vi "Process.vi"(8 "error in":errorcluster, 11 "Example Instrument":refnum<class "Example Instrument.lvclass">) -> (0 "error out":errorcluster, 3 "Example Instrument out":refnum<class "Example Instrument.lvclass">)   [LabVIEW 2016, in "Example Instrument.lvclass"]
doc: "---------------------------------------------------------------\nJKI State Machine Objects™\nhttp://jki.net/state-machine-objects/\nCopyright (C) 2005-2015, JKI <info@jki.net>\nALL RIGHTS RESERVED"
uses:
  Example Instrument.lvclass
  C:/Program Files (x86)/National Instruments/LabVIEW 2016/vi.lib/JKI/JKI SMO/SMO/SMO.lvclass
  <vilib>/JKI/JKI SMO/SMO/Typedefs/Parent Call--Enum.ctl
  Typedefs/PrivateEvents--Example Instrument.setMagnet.ctl
  RemoteControl/RemoteControl.lvclass
  Instrument/Instrument.lvclass
  <vilib>/JKI/JKI SMO/SMO/SMO.lvclass
panel:
  # "Example INSTRUMENT"
  # "For instructions on how to use the JKI State Machine Objects, examples and video tutorials, visit:\nhttp://jki.net/state-machine-objects/\n\nJKI State Machine Objects™\nhttp://jki.net/state-machine-objects/\nCopyright (C) 2005-2015, JKI <info@jki.net>\nALL RIGHTS RESERVED"
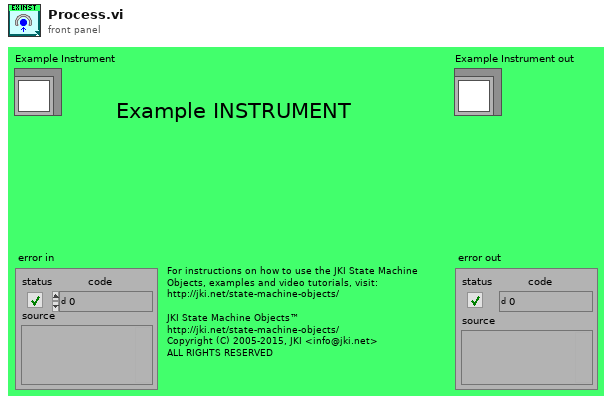
[diagram p1: front panel]
types:
  T1 = typedef "SMO.lvclass/Parent Call--Enum.ctl" = enum16{"Allows parent to run", "Does not request parent to run"}
  T2 = enum32{"invalid app kind", "Development System", "Run Time System", "Student Edition", "Embedded LabVIEW", "Evaluation", "Custom"}
  T3 = enum32{"Invalid", "Standard", "Closed", "Hidden", "Minimized", "Maximized"}
  T4 = enum32{"Bad", "Idle", "Run top level", "Running"}
  T5 = typedef "Example Instrument.lvclass/PrivateEvents--Example Instrument.setMagnet.ctl" = cluster{"setMagnet":dbl, "notifier":refnum<notifier>}
  T6 = cluster{"Core":cluster{"Current VI Reference":refnum<vi>, "Close Panel on Exit?":bool, "error":errorcluster}, "Self Reference":refnum<class "Example Instrument.lvclass">, "setMagnet":T5, "RemoteControl.lvclass":refnum<class "RemoteControl.lvclass">}
  T7 = cluster{"Current VI Reference":refnum<vi>, "Close Panel on Exit?":bool, "error":errorcluster}
  T8 = typedef "SMO.lvclass/Protected Events.ctl" = cluster{"StopProcesses":refnum<user-event>, "AbortProcesses":refnum<user-event>, "Config Changed":refnum<user-event>, "Dependency":refnum<user-event>}
  T9 = typedef "Example Instrument.lvclass/PrivateEvents--Cluster.ctl" = cluster{"setMagnet":refnum<user-event>}
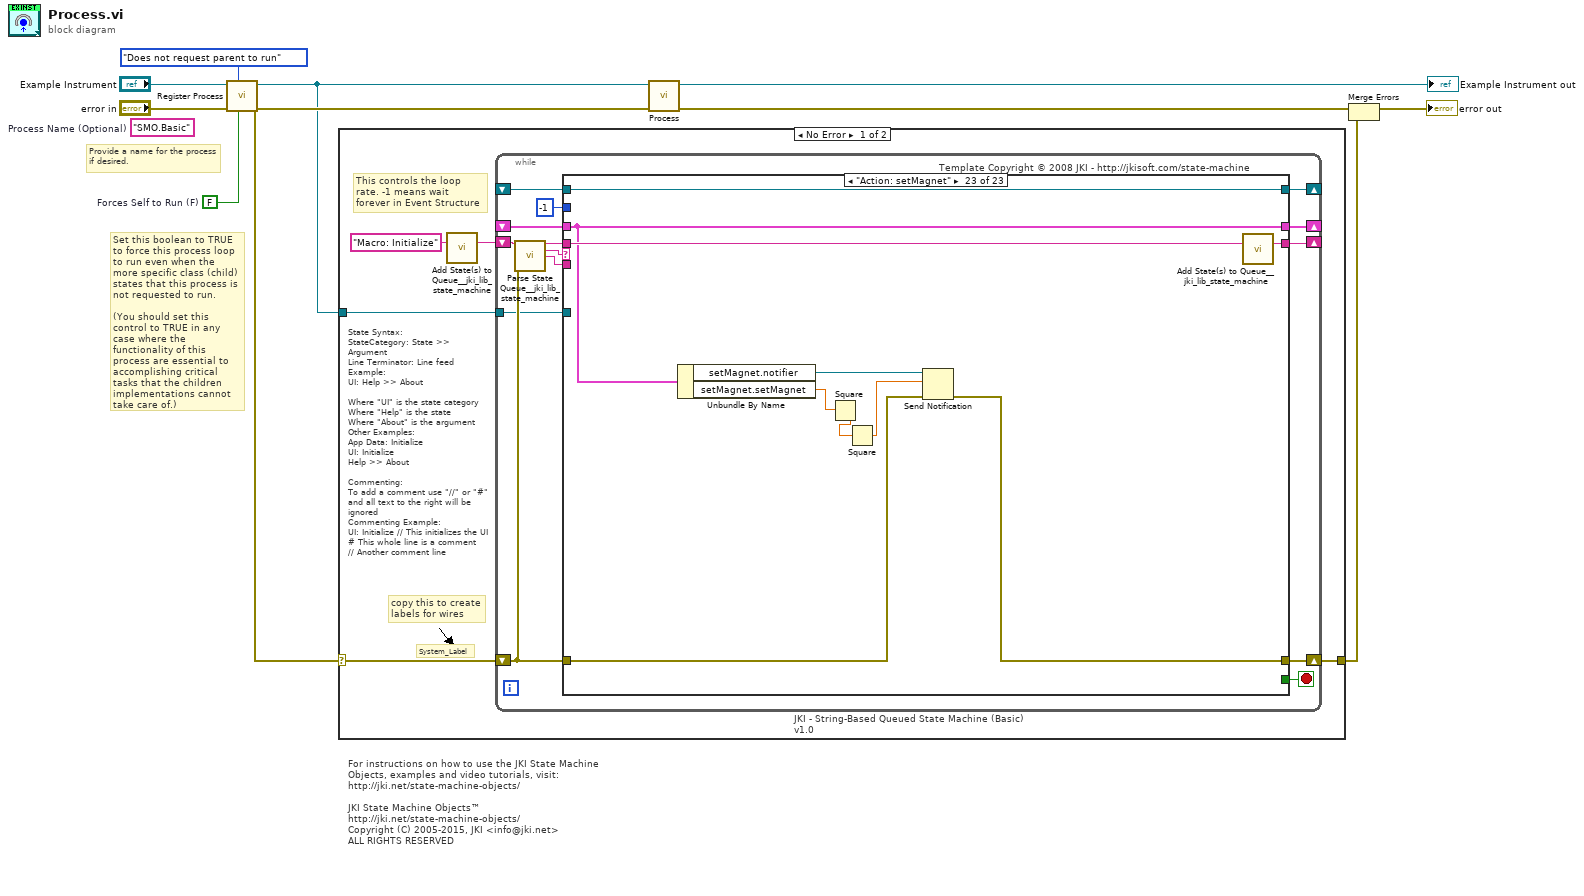
[diagram p0: block diagram]
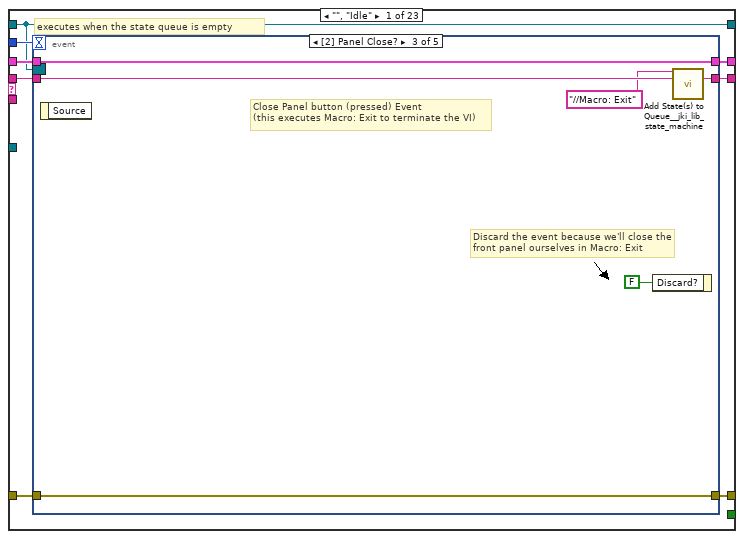
[diagram p2: hidden frame]
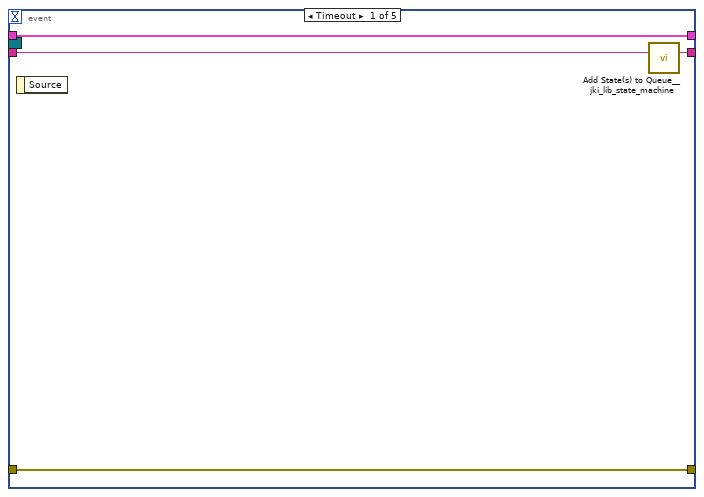
[diagram p3: hidden frame]
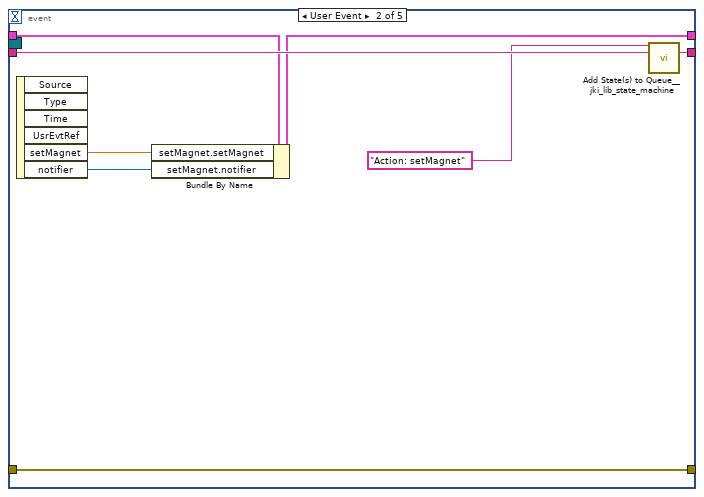
[diagram p4: hidden frame]
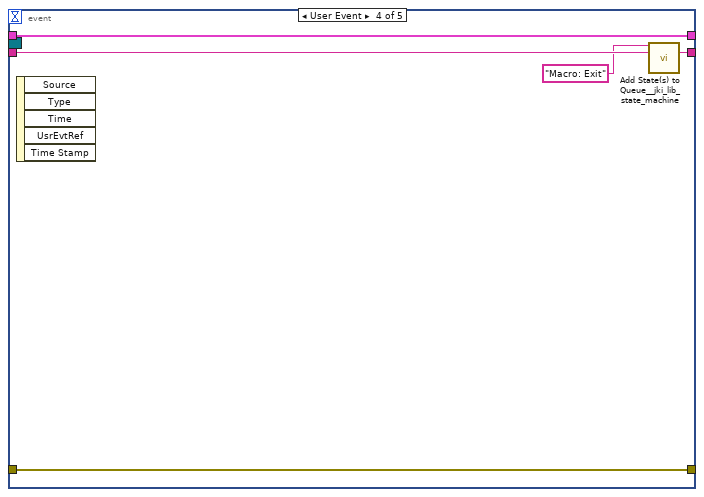
[diagram p5: hidden frame]
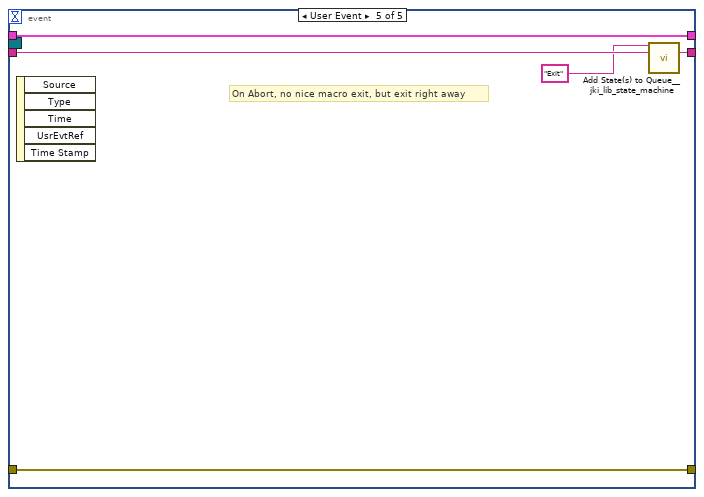
[diagram p6: hidden frame]
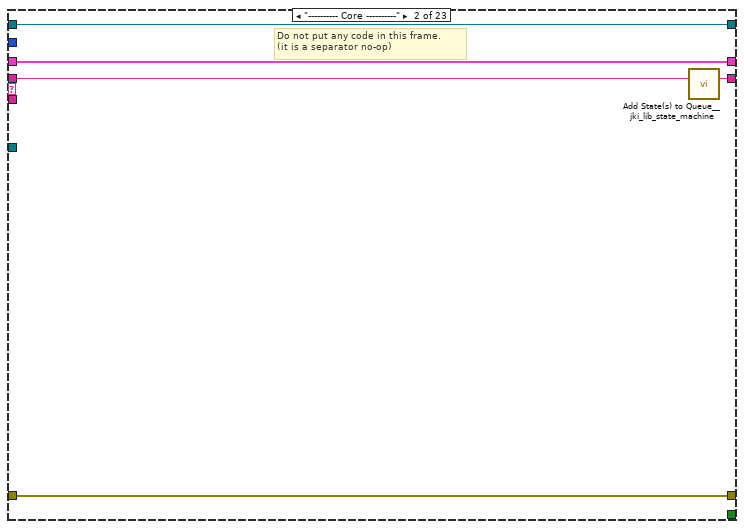
[diagram p7: hidden frame]
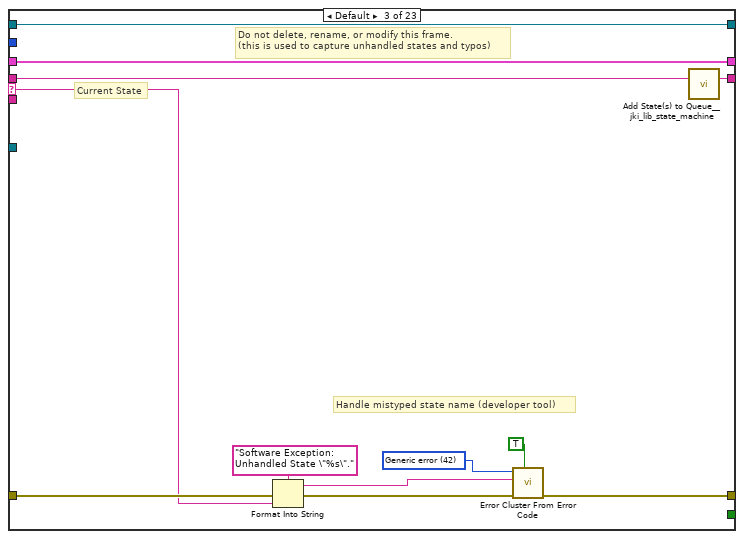
[diagram p8: hidden frame]
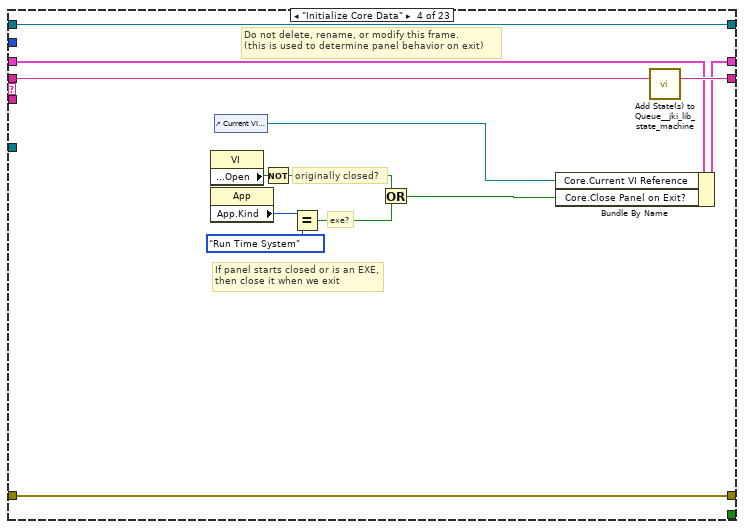
[diagram p9: hidden frame]
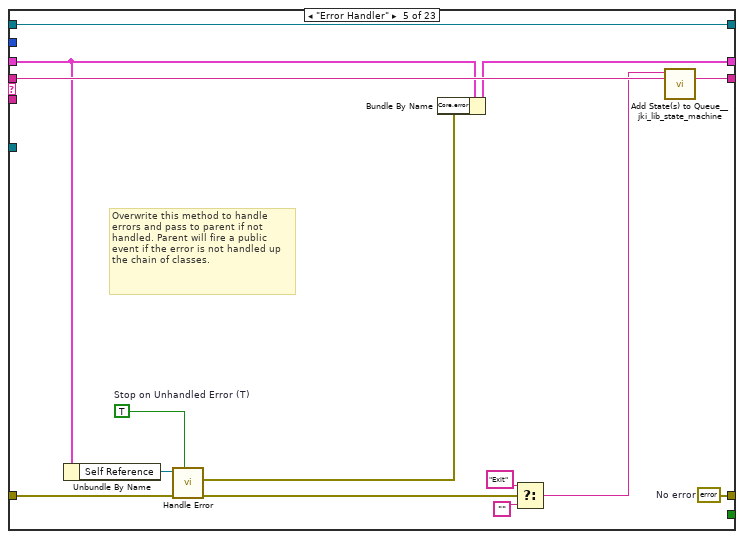
[diagram p10: hidden frame]
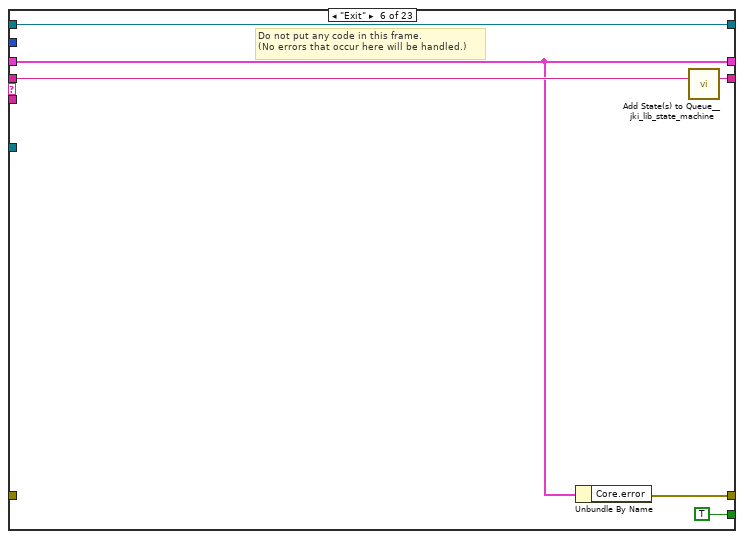
[diagram p11: hidden frame]
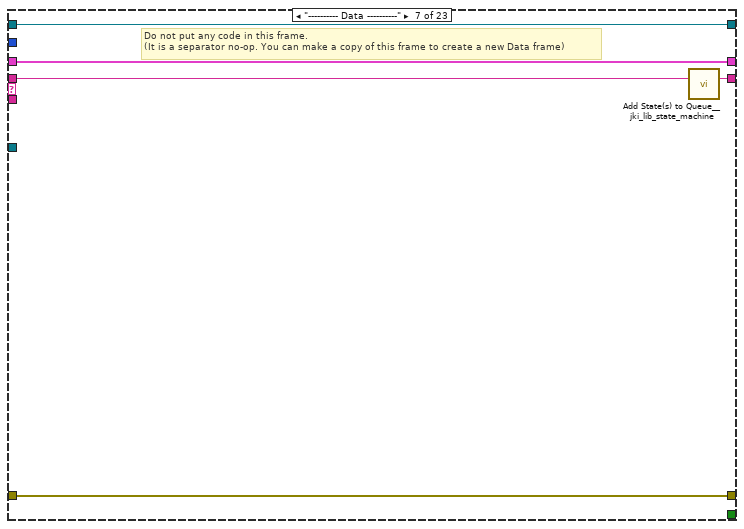
[diagram p12: hidden frame]
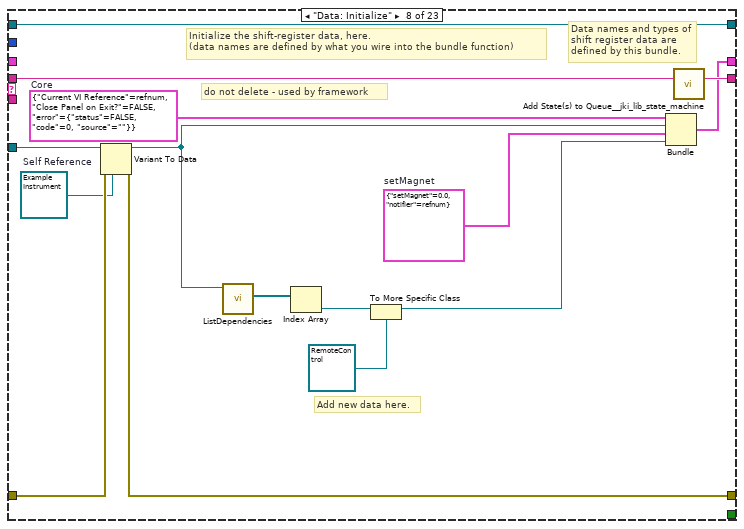
[diagram p13: hidden frame]
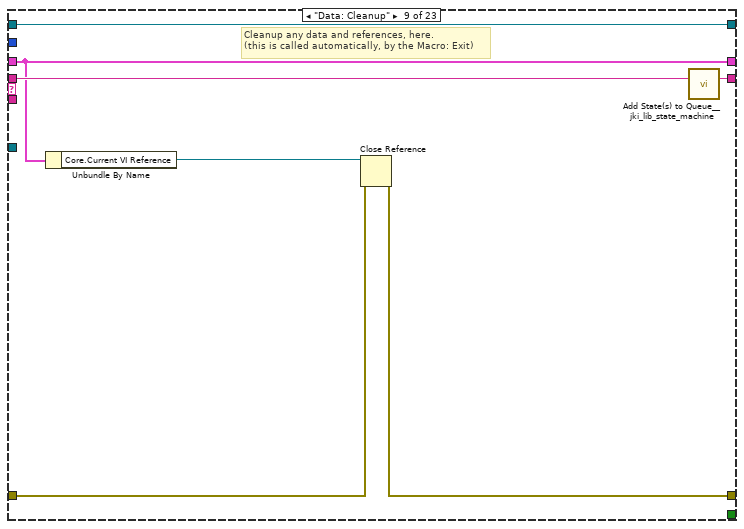
[diagram p14: hidden frame]
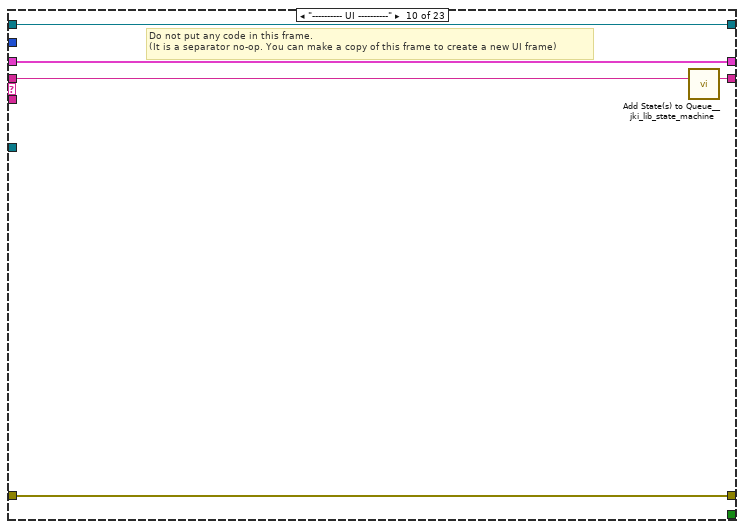
[diagram p15: hidden frame]
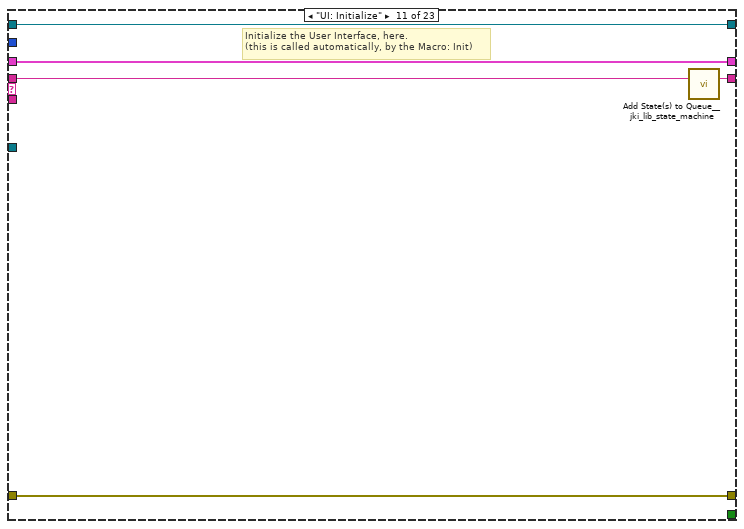
[diagram p16: hidden frame]
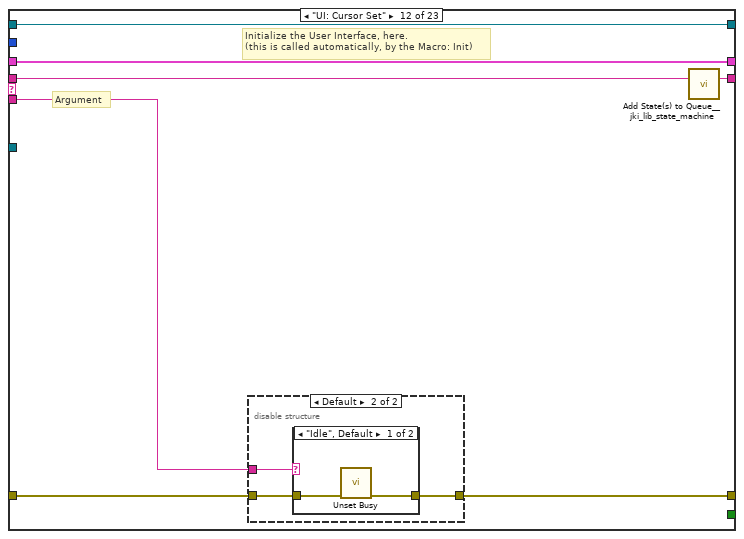
[diagram p17: hidden frame]
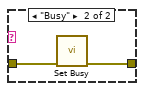
[diagram p19: hidden frame]
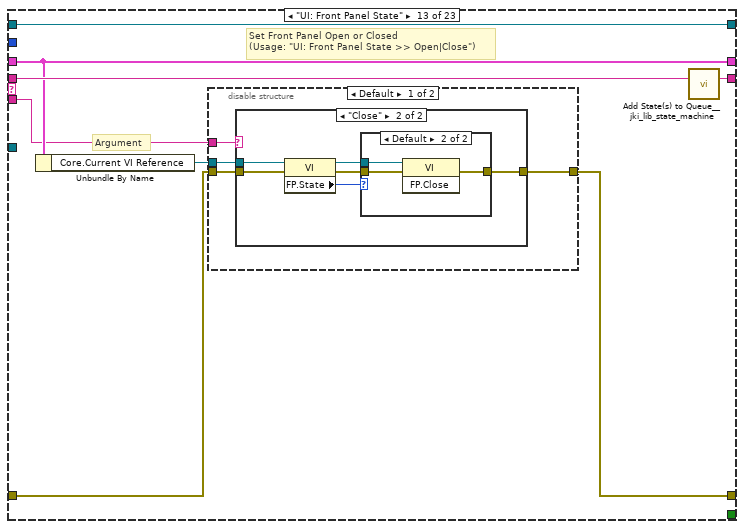
[diagram p20: hidden frame]
diagram:
  w1 = FALSE  # Forces Self to Run (F)
  (unwired) "SMO.Basic"  # Process Name (Optional)
  # "Provide a name for the process\nif desired."
  # "Set this boolean to TRUE to force this process loop to run even when the more specific class (child) states that this process is not requested to run.\n\n(You should set this control to TRUE in any case where the functionality of this process are essential to accomplishing critical tasks that the children implementations cannot take care of.)"
  # "For instructions on how to use the JKI State Machine Objects, examples and video tutorials, visit:\nhttp://jki.net/state-machine-objects/\n\nJKI State Machine Objects™\nhttp://jki.net/state-machine-objects/\nCopyright (C) 2005-2015, JKI <info@jki.net>\nALL RIGHTS RESERVED"
  n1 = call <vilib>:"Register Process.vi"("Forces Self to Run (F)"=w1, "Parent Call"=Parent_Call--Enum."Does not request parent to run", "error in (no error)"="error in", "SMO"="Example Instrument") -> ("error out"=w7:errorcluster, "SMO out"=w6:refnum<class "Example Instrument.lvclass">)  [unwired: 6 in]
  n2 = case shown="No Error" w7 {
    selector: w7 -> [w12 w289]
    tunnel: w6 -> [w13 _]
    tunnel: [w11 w289] -> w3
    frame No Error {
      # "State Syntax:\nStateCategory: State >> Argument\nLine Terminator: Line feed\nExample:\nUI: Help >> About\n\nWhere \"UI\" is the state category\nWhere \"Help\" is the state\nWhere \"About\" is the argument\nOther Examples:\nApp Data: Initialize\nUI: Initialize\nHelp >> About\n\nCommenting:\nTo add a comment use \"//\" or \"#\" and all text to the right will be ignored\nCommenting Example:\nUI: Initialize // This initializes the UI\n# This whole line is a comment\n// Another comment line"
      # "copy this to create labels for wires"
      # "This controls the loop rate. -1 means wait forever in Event Structure"
      # "System_Label"
      n3 = call <vilib>:"Add State(s) to Queue__jki_lib_state_machine.vi"("State(s) in (\"\")"="Macro: Initialize") -> ("States Out"=w15:string)  [unwired: 14 in]
      n4 = while "JKI - String-Based Queued State Machine (Basic) v1.0" {
        shift-right: [w22] -> _
        shift-left: _ -> [w21]
        shift-right: [w25] -> w11
        shift-left: w12 -> [w19]
        shift-right: [w24] -> _
        shift-left: w15 -> [w26]
        tunnel: w13 -> [w18]
        shift-right: [w17] -> _
        shift-left: _ -> [w16]
        stop <- w23 stop-if-true
        # "Template Copyright © 2008 JKI - http://jkisoft.com/state-machine"
        n5 = call <vilib>:"Parse State Queue__jki_lib_state_machine.vi"("State Queue"=w26, "Error In (no error)"=w19) -> ("Remaining States"=w28:string, "Current State"=w29:string, "Arguments"=w27:string)  [unwired: 11 in]
        n6 = case shown="\"Action: setMagnet\"" w29 {
          selector: w29 -> [_ _ w72 _ _ _ _ _ _ _ _ _ _ _ _ _ _ _ _ _ _ _ _]
          tunnel: w28 -> [w37 w70 w76 w95 w109 w115 w120 w135 w142 w147 w152 w159 w175 w207 w221 w235 w240 w251 w256 w267 w273 w278 w288]
          tunnel: w27 -> [_ _ _ _ _ _ _ _ _ _ _ w153 w169 _ _ _ _ _ _ _ _ _ _]
          tunnel: w21 -> [w35 w67 w74 w86 w103 w111 w117 _ w137 w144 w150 w157 w171 w204 w217 w226 w237 w248 w253 w257 w271 w276 w285]
          tunnel: [w34 w68 w78 w92 w104 w110 w118 w131 w138 w145 w149 w154 w172 w205 w219 w233 w238 w242 w254 w262 w269 w274 w282] -> w25
          tunnel: w19 -> [w33 w68 w77 w92 w105 _ w118 w132 w139 w145 w149 w155 w173 w205 w219 w233 w238 w243 w254 w263 w269 w274 w283]
          tunnel: [w36 w69 w75 w94 w108 w114 w119 w134 w141 w146 w151 w158 w174 w206 w220 w234 w239 w250 w255 w266 w272 w277 w287] -> w24
          tunnel: [_ _ _ _ _ TRUE _ _ _ _ _ _ _ _ _ _ _ _ _ _ _ _ _] -> w23
          tunnel: [w32 w67 w74 w93 w102 w111 w117 w133 w137 w144 w150 w157 w171 w204 w217 w226 w237 w248 w253 w257 w271 w276 w285] -> w22
          tunnel: -1 ("Timeout") -> [w31 _ _ _ _ _ _ _ _ _ _ _ _ _ _ _ _ _ _ _ _ _ _]
          tunnel: w18 -> [_ _ _ _ _ _ _ w129 _ _ _ _ _ _ _ _ _ _ _ _ _ _ _]
          tunnel: [w30 w66 w71 w83 w107 w112 w116 w128 w136 w143 w148 w156 w168 w203 w218 w227 w236 w249 w252 w265 w270 w275 w286] -> w17
          tunnel: w16 -> [w30 w66 w71 w83 w107 w112 w116 w128 w136 w143 w148 w156 w168 w203 w218 w227 w236 w249 w252 _ w270 w275 w286]
          frame "", "Idle" {
            # "executes when the state queue is empty"
            n7 = event shown="[2] Panel Close?" {
              selector: w30 -> [_ _ _ _ _]
              dyn-events: _ -> [_ _ _ _ _]
              timeout: w31 -> [_ _ _ _ _]
              tunnel: w37 -> [w41 w49 w55 w60 w65]
              tunnel: [w40 w48 w54 w59 w64] -> w36
              tunnel: w35 -> [w38 w43 w52 w57 w62]
              tunnel: [w39 w47 w53 w58 w63] -> w34
              tunnel: w33 -> [w39 w47 w53 w58 w63]
              tunnel: [w38 w42 w52 w57 w62] -> w32
              event Timeout {
                n8 = event-data() -> ()  [unwired: 1 in, 1 out]
                n9 = call <vilib>:"Add State(s) to Queue__jki_lib_state_machine.vi"("State(s) in (\"\")"=w41) -> ("States Out"=w40:string)  [unwired: 14 in]
              }
              event User Event {
                n10 = event-data() -> ("setMagnet"=w45:dbl, "notifier"=w44:refnum<notifier>)  [unwired: 1 in, 4 out]
                n11 = Bundle By Name(cluster=w43, "setMagnet.setMagnet"=w45, "setMagnet.notifier"=w44) -> (w42:T6)
                n12 = call <vilib>:"Add State(s) to Queue__jki_lib_state_machine.vi"("State(s) in Front (\"\")"="Action: setMagnet" ("State(s) in Front (\"\")"), "State(s) in (\"\")"=w49) -> ("States Out"=w48:string)  [unwired: 13 in]
              }
              event Panel Close? {
                # "Discard the event because we'll close the front panel ourselves in Macro: Exit"
                # "Close Panel button (pressed) Event\n(this executes Macro: Exit to terminate the VI)"
                n13 = event-data() -> ()  [unwired: 1 in, 1 out]
                n14 = event-data("Discard?"=FALSE) -> ()  [unwired: 1 in, 1 out]
                n15 = call <vilib>:"Add State(s) to Queue__jki_lib_state_machine.vi"("State(s) in Front (\"\")"="//Macro: Exit", "State(s) in (\"\")"=w55) -> ("States Out"=w54:string)  [unwired: 13 in]
              }
              event User Event {
                n16 = event-data() -> ()  [unwired: 1 in, 5 out]
                n17 = call <vilib>:"Add State(s) to Queue__jki_lib_state_machine.vi"("State(s) in Front (\"\")"="Macro: Exit", "State(s) in (\"\")"=w60) -> ("States Out"=w59:string)  [unwired: 13 in]
              }
              event User Event {
                # "On Abort, no nice macro exit, but exit right away"
                n18 = event-data() -> ()  [unwired: 1 in, 5 out]
                n19 = call <vilib>:"Add State(s) to Queue__jki_lib_state_machine.vi"("State(s) in Front (\"\")"="Exit", "State(s) in (\"\")"=w65) -> ("States Out"=w64:string)  [unwired: 13 in]
              }
            }
          }
          frame "---------- Core ----------" {
            # "Do not put any code in this frame.\n(it is a separator no-op)"
            n20 = call <vilib>:"Add State(s) to Queue__jki_lib_state_machine.vi"("State(s) in (\"\")"=w70) -> ("States Out"=w69:string)  [unwired: 14 in]
          }
          frame Default {
            w81 = 42 items=["No error", "Argument error", "Memory is full", "Out of zone", "End of file", "File already open", "Generic file I/O error", "File not found", "File permission error", "Disk is full", "Duplicate path", "Too many files open", "System feature not enabled", "Resource file not found", "Cannot add resource", "Resource not found", "Image not found", "Image memory error", "Pen does not exist", "Config type invalid", "Config token not found", "Config parse error", "Config memory error", "Bad external code format", "Bad external code offset", "External code not present", "Null window", "Destroy window error", "Null menu", "Print aborted", "Bad print record", "Print driver error", "Windows error during printing", "Memory error during printing", "Print dialog error", "Generic print error", "Invalid device refnum", "Device not found", "Device parameter error", "Device unit error", "Cannot open device", "Device call aborted", "Generic error", "Cancelled by user", "Object ID too low", "Object ID too high", "Object not in heap", "Unknown heap", "Unknown object (invalid DefProc)", "Unknown object (DefProc not in table)", "Message out of range", "Invalid (null) method", "Unknown message", "Manager call not supported", "Bad address", "Network operation in progress", "Network operation timed out", "Connection is busy", "Network attribute not supported", "Network error", "Address in use", "System out of memory", "Connection aborted", "Connection refused", "Not connected", "Already connected", "Connection closed", "Initialization error (interapplication manager)", "Bad occurrence", "Wait on unbound occurrence handler", "Occurrence queue overflow", "Datalog type conflict", "Unused", "Unrecognized type (interapplication manager)", "Memory corrupt", "Failed to make temporary DLL", "Old CIN version", "Drag socket not found", "Failed to load drop-object", "Failed to register OLE object", "Failed to release OLE object", "Format specifier type mismatch", "Unknown format specifier", "Too few format specifiers", "Too many format specifiers", "Scan failed", "Newer CIN version", "Error converting to variant", "Runtime menu error", "Password tampered", "Variant attribute not found", "Incompatible variant data type", "Event data is not available", "Event Store is not present", "Occurrence is not found", "Event Queue is not created", "Event info is not available", "Refnum passed is NULL", "Error retrieving Class GUID", "Error retrieving CoClass GUID", "Error retrieving TypeLib GUID.", "Bad built application magic bytes.", "Specific driver is different from the specific driver associated with the Logical Name.", "There is no session opened to the class driver.", "Max Error", "MAX - Error with config objects", "MAX - Error loading configuration", "MAX - Group not supported"]
            # "Current State"
            # "Do not delete, rename, or modify this frame.\n(this is used to capture unhandled states and typos)"
            # "Handle mistyped state name (developer tool)"
            n21 = Format Into String(format string="Software Exception: Unhandled State \"%s\"." ("message"), error in=w77, w72) -> (resulting string=w80:string, error out=w79:errorcluster)  [unwired: 1 in]
            n22 = call <vilib>:"Error Cluster From Error Code.vi"("show call chain? (False)"=TRUE, "error in (no error)"=w79, "error message (\"\")"=w80, "error code (0)"=w81) -> ("error out"=w78:errorcluster)  [unwired: 5 in]
            n23 = call <vilib>:"Add State(s) to Queue__jki_lib_state_machine.vi"("State(s) in (\"\")"=w76) -> ("States Out"=w75:string)  [unwired: 14 in]
          }
          frame "Initialize Core Data" {
            # "Do not delete, rename, or modify this frame.\n(this is used to determine panel behavior on exit)"
            # "originally closed?"
            # "exe?"
            # "If panel starts closed or is an EXE, then close it when we exit"
            n24 = property class="VI"() -> ("Front Panel.Open"=w91:bool)  [unwired: 2 in, 2 out]
            n25 = property class="App"() -> ("App.Kind"=w90:T2)  [unwired: 2 in, 2 out]
            n26 = control-ref of="Current VI Reference"() -> (w84:refnum<vi>)
            n27 = Not(x=w91) -> (.not. x?=w88:bool)
            n28 = Equal?(x=w90, y=T2."Run Time System" ("Application:Kind")) -> (x = y?=w87:bool)
            n29 = Or(x=w88, y=w87) -> (x .or. y?=w85:bool)
            n30 = Bundle By Name(cluster=w86, "Core.Current VI Reference"=w84, "Core.Close Panel on Exit?"=w85) -> (w93:T6)
            n31 = call <vilib>:"Add State(s) to Queue__jki_lib_state_machine.vi"("State(s) in (\"\")"=w95) -> ("States Out"=w94:string)  [unwired: 14 in]
          }
          frame "Error Handler" {
            w96 = TRUE  # Stop on Unhandled Error (T)
            w104 = errorcluster {"status"=FALSE, "code"=0, "source"=""}  # No error
            # "Overwrite this method to handle errors and pass to parent if not handled. Parent will fire a public event if the error is not handled up the chain of classes."
            n32 = Unbundle By Name(w103) -> ("Self Reference"=w106:refnum<class "Example Instrument.lvclass">)
            n33 = call-dynamic "Handle Error.vi"("Stop on Unhandled Error (T)"=w96, "error in"=w105, "LevyLab"=w106) -> ("handling error"=w97:errorcluster, "Unhandled error"=w100:errorcluster)  [unwired: 6 in, 1 out]
            n34 = Bundle By Name(cluster=w103, "Core.error"=w100) -> (w102:T6)
            n35 = Select(t="Exit", s=w97, f="") -> (s? t:f=w101:string)
            n36 = call <vilib>:"Add State(s) to Queue__jki_lib_state_machine.vi"("State(s) in Front (\"\")"=w101, "State(s) in (\"\")"=w109) -> ("States Out"=w108:string)  [unwired: 13 in]
          }
          frame "Exit" {
            # "Do not put any code in this frame.\n(No errors that occur here will be handled.)"
            n37 = Unbundle By Name(w111) -> ("Core.error"=w110:errorcluster)
            n38 = call <vilib>:"Add State(s) to Queue__jki_lib_state_machine.vi"("State(s) in (\"\")"=w115) -> ("States Out"=w114:string)  [unwired: 14 in]
          }
          frame "---------- Data ----------" {
            # "Do not put any code in this frame.\n(It is a separator no-op. You can make a copy of this frame to create a new Data frame)"
            n39 = call <vilib>:"Add State(s) to Queue__jki_lib_state_machine.vi"("State(s) in (\"\")"=w120) -> ("States Out"=w119:string)  [unwired: 14 in]
          }
          frame "Data: Initialize" {
            w126 = T5 {"setMagnet"=0.0, "notifier"=refnum}  # setMagnet
            w127 = T7 {"Current VI Reference"=refnum, "Close Panel on Exit?"=FALSE, "error"={"status"=FALSE, "code"=0, "source"=""}}  # Core
            w130 = refnum<class "Example Instrument.lvclass"> refnum  # Self Reference
            # "do not delete - used by framework"
            # "Add new data here."
            # "Data names and types of shift register data are defined by this bundle."
            # "Initialize the shift-register data, here.\n(data names are defined by what you wire into the bundle function)"
            n40 = Variant To Data(error in=w132, type=w130, Variant=w129) -> (data=w121:refnum<class "Example Instrument.lvclass">, error out=w131:errorcluster)
            n41 = call <vilib>:"ListDependencies.vi"("SMO in"=w121) -> ("[Dependencies]"=w125:refnum<class "SMO.lvclass">[])  [unwired: 7 in, 3 out]
            n42 = Index Array(array=w125) -> (element=w124:refnum<class "SMO.lvclass">)  [unwired: 1 in]
            n43 = To More Specific Class(target class=refnum<class "RemoteControl.lvclass"> refnum ("RemoteControl.lvclass"), reference=w124) -> (specific class reference=w123:refnum<class "RemoteControl.lvclass">)  [unwired: 1 in, 1 out]
            n44 = Bundle("Core"=w127, "Self Reference"=w121, "setMagnet"=w126, "RemoteControl.lvclass"=w123) -> (w133:T6)  [unwired: 1 in]
            n45 = call <vilib>:"Add State(s) to Queue__jki_lib_state_machine.vi"("State(s) in (\"\")"=w135) -> ("States Out"=w134:string)  [unwired: 14 in]
          }
          frame "Data: Cleanup" {
            # "Cleanup any data and references, here.\n(this is called automatically, by the Macro: Exit)"
            n46 = Unbundle By Name(w137) -> ("Core.Current VI Reference"=w140:refnum<vi>)
            n47 = Close Reference(reference=w140, error in (no error)=w139) -> (error out=w138:errorcluster)
            n48 = call <vilib>:"Add State(s) to Queue__jki_lib_state_machine.vi"("State(s) in (\"\")"=w142) -> ("States Out"=w141:string)  [unwired: 14 in]
          }
          frame "---------- UI ----------" {
            # "Do not put any code in this frame.\n(It is a separator no-op. You can make a copy of this frame to create a new UI frame)"
            n49 = call <vilib>:"Add State(s) to Queue__jki_lib_state_machine.vi"("State(s) in (\"\")"=w147) -> ("States Out"=w146:string)  [unwired: 14 in]
          }
          frame "UI: Initialize" {
            # "Initialize the User Interface, here.\n(this is called automatically, by the Macro: Init)"
            n50 = call <vilib>:"Add State(s) to Queue__jki_lib_state_machine.vi"("State(s) in (\"\")"=w152) -> ("States Out"=w151:string)  [unwired: 14 in]
          }
          frame "UI: Cursor Set" {
            # "Argument"
            # "Initialize the User Interface, here.\n(this is called automatically, by the Macro: Init)"
            n51 = disable-structure shown="Default" {
              disable-tunnel: w155 -> [w160 w163]
              disable-tunnel: [w160 w162] -> w154
              disable-tunnel: w153 -> [_ w161]
              frame condition #0 {
              }
              frame condition #1 (active) {
                n52 = case shown="\"Idle\", Default" w161 {
                  tunnel: w163 -> [w165 w167]
                  tunnel: [w164 w166] -> w162
                  frame "Idle", Default {
                    n53 = call <vilib>:"Unset Busy.vi"("error in (no error)"=w165) -> ("error out"=w164:errorcluster)  [unwired: 10 in]
                  }
                  frame "Busy" {
                    n54 = call <vilib>:"Set Busy.vi"("error in (no error)"=w167) -> ("error out"=w166:errorcluster)  [unwired: 9 in, 1 out]
                  }
                }
              }
            }
            n55 = call <vilib>:"Add State(s) to Queue__jki_lib_state_machine.vi"("State(s) in (\"\")"=w159) -> ("States Out"=w158:string)  [unwired: 14 in]
          }
          frame "UI: Front Panel State" {
            # "Argument"
            # "Set Front Panel Open or Closed\n(Usage: \"UI: Front Panel State >> Open|Close\")"
            n56 = Unbundle By Name(w171) -> ("Core.Current VI Reference"=w170:refnum<vi>)
            n57 = disable-structure shown="Default" {
              disable-tunnel: w173 -> [w179 w202]
              disable-tunnel: [w178 w202] -> w172
              disable-tunnel: w170 -> [w177 _]
              disable-tunnel: w169 -> [w176 _]
              frame condition #0 (active) {
                n58 = case shown="\"Close\"" w176 {
                  tunnel: w179 -> [w183 w196]
                  tunnel: [w185 w197] -> w178
                  tunnel: w177 -> [w184 w194]
                  frame "Open", Default {
                    n59 = property class="VI"(reference=w184, error in=w183) -> (reference out=w181:refnum<vi>, error out=w182:errorcluster, "FP.State"=w180:T3)
                    n60 = case shown="\"Closed\"" w180 {
                      tunnel: [w188 w191] -> w185
                      tunnel: w182 -> [w187 w191]
                      tunnel: w181 -> [w186 _]
                      frame "Closed" {
                        n61 = invoke class="VI" method="FP.Open"(reference=w186, error in=w187, "Activate"=TRUE, "State"=T3."Standard") -> (error out=w188:errorcluster)  [unwired: 1 in, 4 out]
                      }
                      frame Default {
                      }
                    }
                  }
                  frame "Close" {
                    n62 = property class="VI"(reference=w194, error in=w196) -> (reference out=w193:refnum<vi>, error out=w195:errorcluster, "FP.State"=w192:T3)
                    n63 = case shown="Default" w192 {
                      tunnel: [w198 w201] -> w197
                      tunnel: w195 -> [w198 w200]
                      tunnel: w193 -> [_ w199]
                      frame "Invalid", "Closed" {
                      }
                      frame Default {
                        n64 = invoke class="VI" method="FP.Close"(reference=w199, error in=w200) -> (error out=w201:errorcluster)  [unwired: 1 in, 2 out]
                      }
                    }
                  }
                }
              }
              frame condition #1 {
              }
            }
            n65 = call <vilib>:"Add State(s) to Queue__jki_lib_state_machine.vi"("State(s) in (\"\")"=w175) -> ("States Out"=w174:string)  [unwired: 14 in]
          }
          frame "---------- Macro ----------" {
            # "Do not put any code in this frame.\n(It is a separator no-op. You can make a copy of this frame to create a new Macro frame)"
            n66 = call <vilib>:"Add State(s) to Queue__jki_lib_state_machine.vi"("State(s) in (\"\")"=w207) -> ("States Out"=w206:string)  [unwired: 14 in]
          }
          frame "Macro: Initialize" {
            w212 = "UI: Initialize\nUI: Front Panel State >> Open"  # UI: Initialize UI: Front Panel State >> Open
            w208 = "Process: Sync"
            # "Initialization Macro\n(This is called once, when the VI starts)"
            n67 = control-ref of="This VI"() -> (w210:refnum<vi>)
            n68 = property class="VI"(reference=w210) -> ("Exec.State"=w209:T4)  [unwired: 1 in, 2 out]
            n69 = Equal?(x=w209, y=T4."Run top level") -> (x = y?=w215:bool)
            n70 = Select(t=w208, s=w215, f="") -> ()  [unwired: 1 out]
            n71 = call <vilib>:"Add State(s) to Queue__jki_lib_state_machine.vi"("State(s) in Front (\"\")"="Data: Initialize\nInitialize Core Data\nEvents: Register", "State(s) in (\"\")"=w208, "State(s) at Back (\"\")"=w212) -> ("States Out"=w211:string)  [unwired: 12 in]
            n72 = call <vilib>:"Add State(s) to Queue__jki_lib_state_machine.vi"("State(s) in Front (\"\")"=w211, "State(s) in (\"\")"=w221) -> ("States Out"=w220:string)  [unwired: 13 in]
          }
          frame "Macro: Exit" {
            # "Exit Macro\n(This is called once, when the VI exits)"
            n73 = Unbundle By Name(w226) -> ("Core.Close Panel on Exit?"=w232:bool)
            n74 = Select(t="UI: Front Panel State >> Close", s=w232, f="") -> (s? t:f=w229:string)
            n75 = call <vilib>:"Add State(s) to Queue__jki_lib_state_machine.vi"("State(s) in Front (\"\")"="Data: Cleanup\nEvents: Unregister", "State(s) in (\"\")"="Process: Sync", "State(s) at Back (\"\")"="Exit") -> ("States Out"=w223:string)  [unwired: 12 in]
            n76 = call <vilib>:"Add State(s) to Queue__jki_lib_state_machine.vi"("State(s) in (\"\")"=w229, "State(s) at Back (\"\")"=w223) -> ("States Out"=w228:string)  [unwired: 13 in]
            n77 = call <vilib>:"Add State(s) to Queue__jki_lib_state_machine.vi"("State(s) in Front (\"\")"=w228, "State(s) in (\"\")"=w235) -> ("States Out"=w234:string)  [unwired: 13 in]
          }
          frame "---------- Process ----------" {
            # "Template Separator\n(You can make a copy of, or modify, this frame)"
            n78 = call <vilib>:"Add State(s) to Queue__jki_lib_state_machine.vi"("State(s) in (\"\")"=w240) -> ("States Out"=w239:string)  [unwired: 14 in]
          }
          frame "Process: Sync" {
            n79 = Unbundle By Name(w248) -> ("Self Reference"=w244:refnum<class "Example Instrument.lvclass">)
            n80 = call <vilib>:"WaitOnProcessSync.vi"("error in (no error)"=w243, "SMO"=w244) -> ("error out"=w242:errorcluster, "Don't run?"=w247:bool)  [unwired: 7 in, 1 out]
            n81 = Select(t="Data: Cleanup\nEvents: Unregister\nExit", s=w247, f="") -> (s? t:f=w241:string)
            n82 = call <vilib>:"Add State(s) to Queue__jki_lib_state_machine.vi"("State(s) in Front (\"\")"=w241, "State(s) in (\"\")"=w251) -> ("States Out"=w250:string)  [unwired: 13 in]
          }
          frame "---------- Events ----------" {
            # "Template Separator\n(You can make a copy of, or modify, this frame)"
            n83 = call <vilib>:"Add State(s) to Queue__jki_lib_state_machine.vi"("State(s) in (\"\")"=w256) -> ("States Out"=w255:string)  [unwired: 14 in]
          }
          frame "Events: Register" {
            # "Expand to add\nmore events"
            n84 = Unbundle By Name(w257) -> ("Self Reference"=w259:refnum<class "Example Instrument.lvclass">)
            n85 = call <vilib>:"GetProtectedEvents.vi"("SMO"=w259) -> ("error out"=w260:errorcluster, "SMO Protected Events"=w264:T8)  [unwired: 8 in, 1 out]
            n86 = call "Example Instrument.GetPrivateEvents.vi"("Example Instrument"=w259) -> ("Private Events"=w258:T9)  [unwired: 8 in, 2 out]
            n87 = register-events(w264, w258) -> (reference out=w265:refnum<event-registration>, error out=w261:errorcluster)  [unwired: 2 in]
            n88 = Merge Errors(w263, w261, w260) -> (w262:errorcluster)
            n89 = call <vilib>:"Add State(s) to Queue__jki_lib_state_machine.vi"("State(s) in (\"\")"=w267) -> ("States Out"=w266:string)  [unwired: 14 in]
          }
          frame "Events: Unregister" {
            n90 = Unregister For Events(event registration refnum=w270, error in=w269) -> (error out=w268:errorcluster)
            n91 = call <vilib>:"Clear Errors.vi"("error in (no error)"=w268) -> ()  [unwired: 5 in, 2 out]
            n92 = call <vilib>:"Add State(s) to Queue__jki_lib_state_machine.vi"("State(s) in (\"\")"=w273) -> ("States Out"=w272:string)  [unwired: 14 in]
          }
          frame "---------- Action ----------" {
            n93 = call <vilib>:"Add State(s) to Queue__jki_lib_state_machine.vi"("State(s) in (\"\")"=w278) -> ("States Out"=w277:string)  [unwired: 14 in]
          }
          frame "Action: setMagnet" {
            n94 = Unbundle By Name(w285) -> ("setMagnet.notifier"=w284:refnum<notifier>, "setMagnet.setMagnet"=w281:dbl)
            n95 = Square(x=w281) -> (x^2=w280:dbl)
            n96 = Square(x=w280) -> (x^2=w279:dbl)
            n97 = Send Notification(notification=w279, notifier=w284, error in (no error)=w283) -> (error out=w282:errorcluster)  [unwired: 1 out]
            n98 = call <vilib>:"Add State(s) to Queue__jki_lib_state_machine.vi"("State(s) in (\"\")"=w288) -> ("States Out"=w287:string)  [unwired: 14 in]
          }
        }
      }
    }
    frame Error {
    }
  }
  n99 = call-parent "Process.vi"("error in"=w7, "Instrument"=w6) -> ("error out"=w4:errorcluster, "Instrument out"=→"Example Instrument out":refnum<class "Example Instrument.lvclass">)  [unwired: 8 in]
  n100 = Merge Errors(w4, w3) -> (→"error out":errorcluster)
